vi "ke37xx Configure Temperature Transducer.vi"(0 "VISA Resource Name":refnum<visa-resource-name>, 7 "Transducer Type":T1(ring), 11 "error in (no error)":errorcluster) -> (4 "VISA Resource Name Out":refnum<visa-resource-name>, 15 "error out":errorcluster)   [LabVIEW 2009, in "Keithley 3700 Series.lvlib"]
doc: "This VI allows you to configure the transducer to use for temperature measurements."
uses:
  <instrlib>/Keithley 3706/Keithley 3700 Series.lvlib
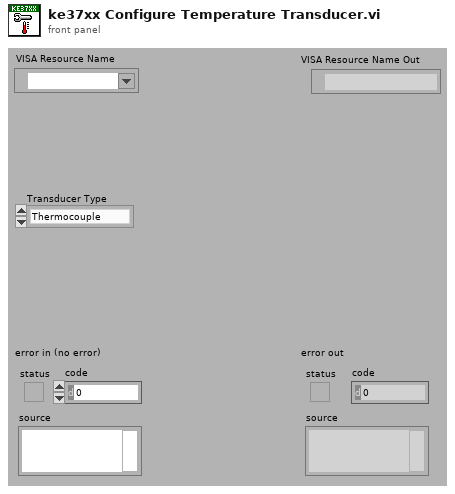
[diagram p1: front panel]
types:
  T1 = enum16{"Thermocouple", "Thermistor", "3-Wire RTD", "4-Wire RTD"}
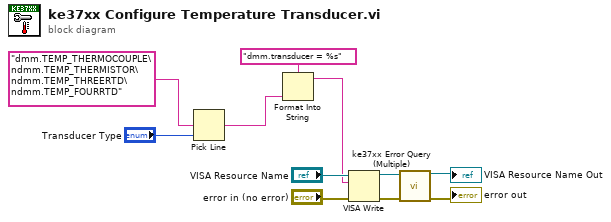
[diagram p0: block diagram]
diagram:
  n1 = Pick Line(multi-line string="dmm.TEMP_THERMOCOUPLE\ndmm.TEMP_THERMISTOR\ndmm.TEMP_THREERTD\ndmm.TEMP_FOURRTD", line index="Transducer Type") -> (output string=w1:string)  [unwired: 1 out]
  n2 = Format Into String(format string="dmm.transducer = %s" ("write buffer"), w1) -> (resulting string=w4:string)  [unwired: 2 in, 1 out]
  n3 = VISA Write(VISA resource name="VISA Resource Name", write buffer=w4, error in (no error)="error in (no error)") -> (VISA resource name out=w7:refnum<visa-resource-name>, error out=w6:errorcluster)  [unwired: 1 out]
  n4 = call <instrlib>:"ke37xx Error Query (Multiple).vi"("VISA resource name"=w7, "error in (no error)"=w6) -> ("VISA resource name out"=→"VISA Resource Name Out":refnum<visa-resource-name>, "error out"=→"error out":errorcluster)  [unwired: 12 out]
